vi "Agilent3446X_Config.vi"(8 "error in":errorcluster caption="错误输入", 11 "MyIndex":u8) -> (0 "error out":errorcluster caption="错误输出", 3 "VISA resource out":refnum<visa-resource-name>)   [LabVIEW 2015]
uses:
  Agilent 3446X Series/Agilent 3446X Series1.lvlib
panel:
  out "OK?":bool
  in  "Manual Resolution":dbl(ring)=1e-05 items=["4.5"=0.0001, "5.5"=1e-05, "6.5"=1e-06]
  in  "Manual Range":dbl=1.0
  in  "量程":bool
  in  "Measurement Function":i32(ring)=10 items=["Continuity", "Current AC", "Current DC", "Diode", "Frequency", "Resistance 4-wire", "Period", "Resistance 2-wire", "Temperature", "Voltage AC", "Voltage DC", "Voltage DC Ratio"]
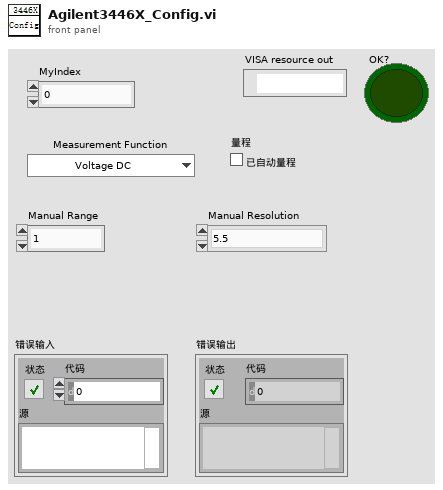
[diagram p1: front panel]
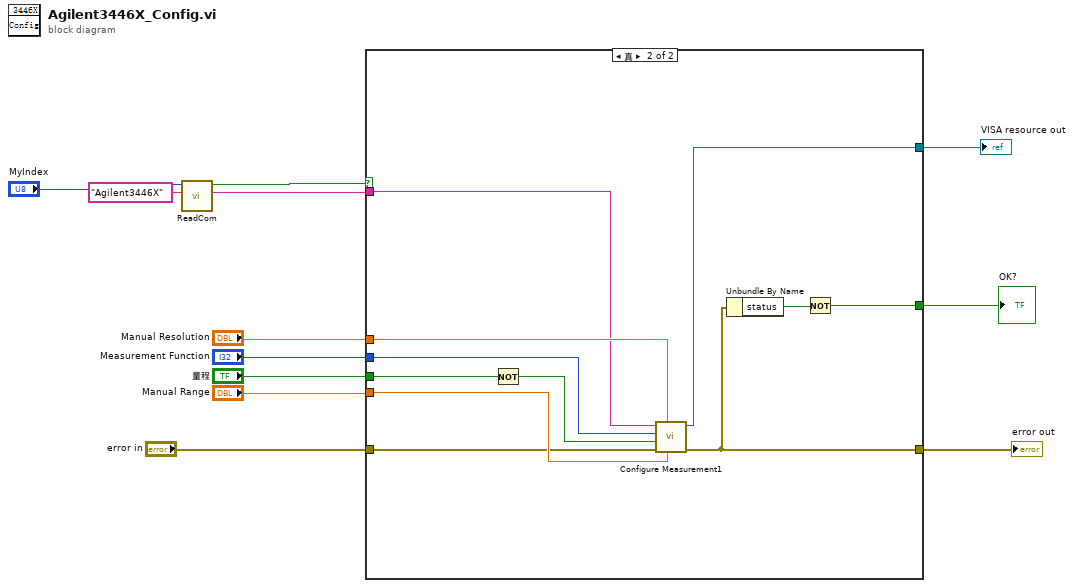
[diagram p0: block diagram]
diagram:
  n1 = call "ReadCom.vi"("仪器名称"="Agilent3446X", "MyIndex"="MyIndex") -> ("COM"=w1:string, "OK?"=w2:bool)  [unwired: 7 in, 1 out]
  n2 = case shown="真" w2 {
    tunnel: [_ w16] -> w12
    tunnel: [_ w23] -> w11
    tunnel: "Measurement Function" -> [_ w22]
    tunnel: "量程" -> [_ w21]
    tunnel: "Manual Range" -> [_ w20]
    tunnel: "Manual Resolution" -> [_ w19]
    tunnel: w1 -> [_ w17]
    tunnel: [_ w14] -> w6
    tunnel: "error in" -> [_ w13]
    frame False {
    }
    frame True {
      n3 = Not(x=w21) -> (.not. x?=w18:bool)
      n4 = call "Configure Measurement1.vi"("Manual Range (1)"=w20, "Absolute Resolution (1E-6)"=w19, "error in (no error)"=w13, "Auto Range (T: Enable)"=w18, "Measurement Function (10: Voltage DC)"=w22, "VISA resource name"=w17) -> ("error out"=w16:errorcluster, "VISA resource name out"=w23:refnum<visa-resource-name>)  [unwired: 4 out]
      n5 = Unbundle By Name(w16) -> ("status"=w15:bool)
      n6 = Not(x=w15) -> (.not. x?=w14:bool)
    }
  }
  "error out" <- w12
  "VISA resource out" <- w11
  "OK?" <- w6
